vi "Execution_StartInternalProcess.vi"(7 "InternalProcess":T1, 8 "error in (no error)":errorcluster, 10 "Process in":refnum<class "Process.lvclass">, 11 "EVE reference in":refnum<data-value>) -> (0 "error out":errorcluster, 3 "EVE reference out":refnum<data-value>)   [LabVIEW 2013, in "Process.lvclass"]
uses:
  Process.lvclass
  EnumProcess.ctl
  001 - MAIN/Class/EVE/EVE.lvclass
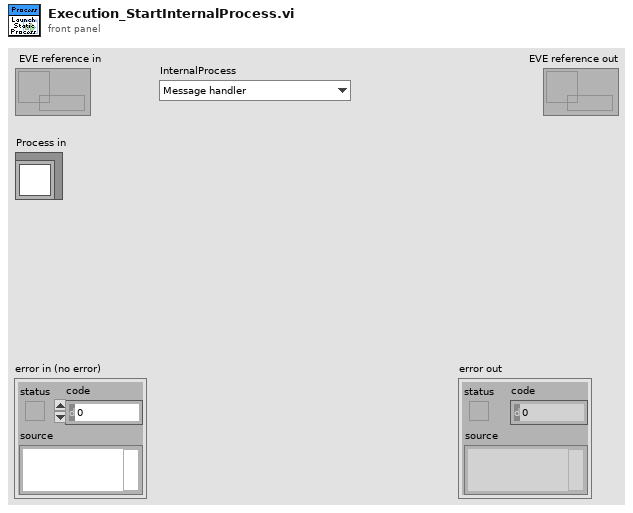
[diagram p1: front panel]
types:
  T1 = typedef "Process.lvclass/EnumProcess.ctl" = enum16{"Message handler", "Template"}
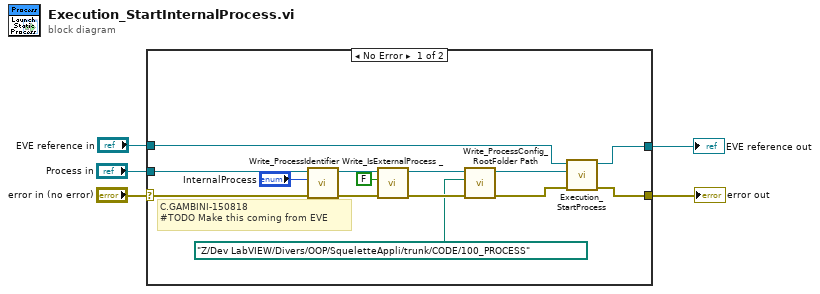
[diagram p0: block diagram]
diagram:
  n1 = case shown="No Error" "error in (no error)" {
    selector: "error in (no error)" -> [w19 w21]
    tunnel: [w18 w21] -> w4
    tunnel: "Process in" -> [w17 _]
    tunnel: "EVE reference in" -> [w16 w20]
    tunnel: [w15 w20] -> w1
    frame No Error {
      # "C.GAMBINI-150818\n#TODO Make this coming from EVE"
      n2 = call-dynamic "Write_ProcessIdentifier.vi"("error in"=w19, "Process"="InternalProcess", "Process in"=w17) -> ("error out"=w12:errorcluster, "Process out"=w13:refnum<class "Process.lvclass">)  [unwired: 7 in]
      n3 = call-dynamic "Write_IsExternalProcess _.vi"("error in (no error)"=w12, "ExternalProcess ?"=FALSE, "Process in"=w13) -> ("error out"=w8:errorcluster, "Process out"=w10:refnum<class "Process.lvclass">)  [unwired: 7 in]
      n4 = call-dynamic "Write_ProcessConfig_RootFolder Path.vi"("error in (no error)"=w8, "RootFolder Path"=path "Z:/Dev LabVIEW/Divers/OOP/SqueletteAppli/trunk/CODE/100_PROCESS", "Process in"=w10) -> ("error out"=w7:errorcluster, "Process out"=w9:refnum<class "Process.lvclass">)  [unwired: 7 in]
      n5 = call "Execution_StartProcess.vi"("error in (no error)"=w7, "Process in"=w9, "EVE reference in"=w16) -> ("error out"=w18:errorcluster, "EVE reference out"=w15:refnum<data-value>)  [unwired: 7 in]
    }
    frame Error {
    }
  }
  "error out" <- w4
  "EVE reference out" <- w1
